vi "SCLN_ReadConfig.vi"(0 "File Path":path, 7 "Section Name":string="AOS", 11 "error in (no error)":errorcluster) -> (8 "IP Info Connection":T1, 15 "error out":errorcluster)   [LabVIEW 2015]
doc: "This VI reads the SOAR Communications Library New configuration file\nand extracts the section name, IP_Server, IP_Client and Ports of system that\nis allowed to connect to this system.\nThe file is a plain ASCII text file with style similar to a windows\n\"*.ini\" file, except that strings like paths are made in a platform\nindependent form."
uses:
  SCLN_InfoClusterConfig.ctl
  <vilib>/Utility/config.llb/NI_LVConfig.lvlib
panel:
  in  "IP Info Template":T1
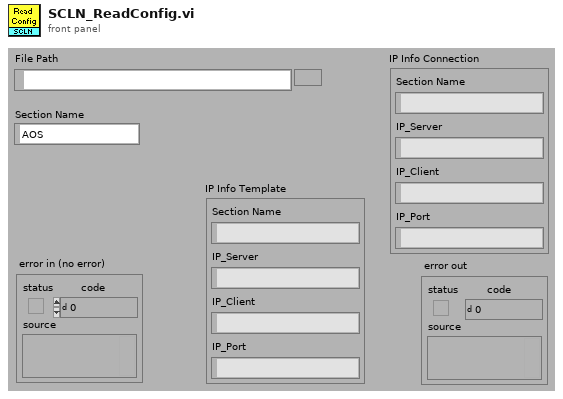
[diagram p1: front panel]
types:
  T1 = typedef "SCLN_InfoClusterConfig.ctl" = cluster{"Section Name":string, "IP_Server":string, "IP_Client":string, "IP_Port":string}
  T2 = typedef "NI_LVConfig.lvlib/Config Data RefNum.ctl" = refnum<k1>
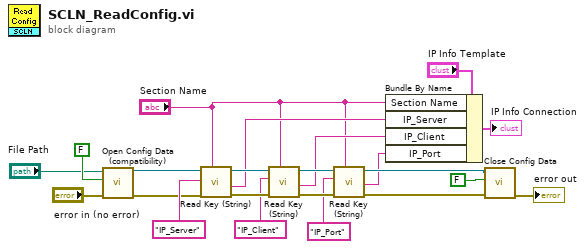
[diagram p0: block diagram]
diagram:
  n1 = call <vilib>:"Open Config Data (compatibility).vi"("error in (no error)"="error in (no error)", "create file if necessary (T)"=FALSE ("create file if necessary? (T)"), "configuration file path"="File Path") -> ("error out"=w1:errorcluster, "refnum"=w2:T2)  [unwired: 6 in, 1 out]
  n2 = call <vilib>:"Read Key (String).vi"("section"="Section Name", "error in (no error)"=w1, "key"="IP_Server", "refnum"=w2) -> ("error out"=w15:errorcluster, "value"=w7:string, "refnum out"=w13:T2)  [unwired: 4 in, 1 out]
  n3 = call <vilib>:"Read Key (String).vi"("section"="Section Name", "error in (no error)"=w15, "key"="IP_Client", "refnum"=w13) -> ("error out"=w17:errorcluster, "value"=w8:string, "refnum out"=w14:T2)  [unwired: 4 in, 1 out]
  n4 = call <vilib>:"Read Key (String).vi"("section"="Section Name", "error in (no error)"=w17, "key"="IP_Port", "refnum"=w14) -> ("error out"=w20:errorcluster, "value"=w9:string, "refnum out"=w19:T2)  [unwired: 4 in, 1 out]
  n5 = Bundle By Name(cluster="IP Info Template", "Section Name"="Section Name", "IP_Server"=w7, "IP_Client"=w8, "IP_Port"=w9) -> (→"IP Info Connection":T1)
  n6 = call <vilib>:"Close Config Data.vi"("error in (no error)"=w20, "write file if changed (T)"=FALSE ("write configuration file? (T)"), "refnum"=w19) -> ("error out"=→"error out":errorcluster)  [unwired: 7 in, 1 out]
